vi "Gear Vision Align.vi"(5 "Reinitialize?":bool, 6 "PID gains":T1={"proportional gain (Kc)"=1.0, "integral time (Ti, min)"=0.01, "derivative time (Td, min)"=0.0} {"derivative time (Td, min)" format="%.3f"; "integral time (Ti, min)" format="%.3f"; "proportional gain (Kc)" format="%.3f"}, 7 "Gyro Tolerance":dbl, 8 "X Min":dbl, 9 "X Max":dbl, 10 "Goal Angle Difference":dbl) -> (0 "Finished?":bool, 3 "X Out":dbl)   [LabVIEW 2016]
uses:
  Common Code/PID Gains.ctl
  Robot Global Data.vi
  <vilib>/addons/control/pid/pid.llb/PID (DBL).vi
  <vilib>/addons/control/pid/NI_PID_pid.lvlib
panel:
  out "Heading Target":dbl
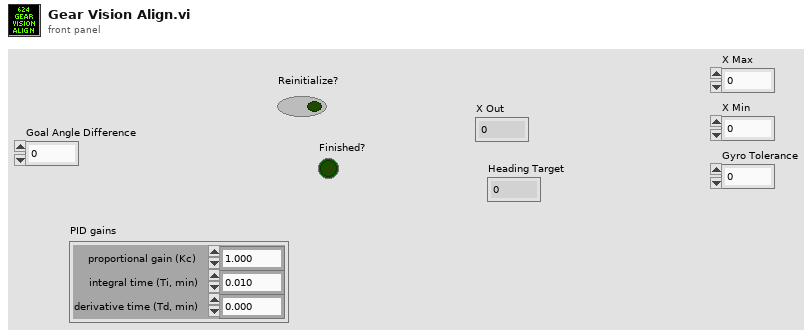
[diagram p1: front panel]
types:
  T1 = typedef "PID Gains.ctl" = cluster{"proportional gain (Kc)":dbl, "integral time (Ti, min)":dbl, "derivative time (Td, min)":dbl}
  T2 = typedef "Drivetrain Status Cluster.ctl" = cluster{"Y (Throttle)":dbl, "X (Steer)":dbl, "Z (Strafe)":dbl, "Heading Target":dbl, "Center Piston Down?":bool, "Traction?":bool, "Gyro Steer Finished?":bool, "Distance Drive Finished?":bool, "Gyro":dbl, "Distance Target":dbl, "Y Max Output":dbl, "Y Min Output":dbl, "X Max Output":dbl, "X Min Output":dbl, "Z Max Output":dbl, "Z Min Output":dbl, "Translation Target":dbl, "Translation Drive Finished?":bool, "PID Auto Drive Finished?":bool, "Brake?":bool, "Vision Aligned?":bool, "Creep Mode Engaged?":bool, "Drivetrain Mode":T3}
  T3 = typedef "Drivetrain Mode.ctl" = enum16{"Gear Vision Align", "Manual", "Gyro Steer", "Distance Drive", "Translate Drive", "Goal Vision Align", "PID Drive"}
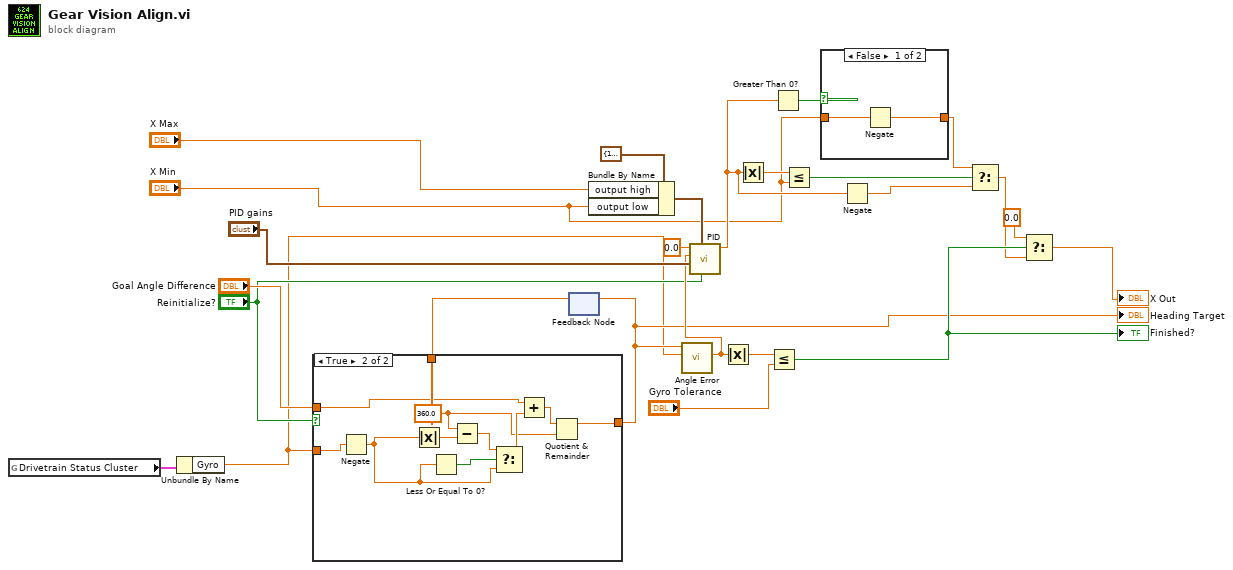
[diagram p0: block diagram]
diagram:
  n1 = global read "Robot Global Data.vi" "Drivetrain Status Cluster"() -> (w11:T2)
  n2 = Unbundle By Name(w11) -> ("Gyro"=w4:dbl)
  n3 = feedback #1() -> (w8:dbl)  [unwired: 1 in]
  n4 = case shown="True" "Reinitialize?" {
    tunnel: [w26 w28] -> w7
    tunnel: "Goal Angle Difference" -> [_ w31]
    tunnel: w8 -> [w26 _]
    tunnel: w4 -> [_ w27]
    frame False {
    }
    frame True {
      w29 = 360.0 ("x")
      n5 = Negate(x=w27) -> (-x=w33:dbl)
      n6 = Absolute Value(x=w33) -> (abs(x)=w35:dbl)
      n7 = Less Or Equal To 0?(x=w33) -> (x <= 0?=w36:bool)
      n8 = Subtract(x=w29, y=w35) -> (x-y=w34:dbl)
      n9 = Select(t=w34, s=w36, f=w33) -> (s? t:f=w32:dbl)
      n10 = Add(x=w31, y=w32) -> (x+y=w30:dbl)
      n11 = Quotient & Remainder(x=w30, y=w29) -> (x-y*floor(x/y)=w28:dbl)  [unwired: 1 out]
    }
  }
  "Heading Target" <- w7
  n12 = feedback-in #1(w7) -> ()
  n13 = Bundle By Name(cluster=cluster{"output high":dbl, "output low":dbl} {"output high"=100.0, "output low"=-100.0} ("output range"), "output high"="X Max", "output low"="X Min") -> (w22:cluster{"output high":dbl, "output low":dbl})
  n14 = call "Angle Error.vi"("Angle"=w4, "Target Angle"=w7) -> ("Error"=w9:dbl)  [unwired: 9 in]
  n15 = call-poly <vilib>:"PID.vi"("reinitialize? (F)"="Reinitialize?", "output range"=w22, "PID gains"="PID gains", "process variable"=w9, "setpoint"=0.0) -> ("output"=w19:dbl)  [unwired: 5 in, 1 out]
  n16 = Absolute Value(x=w9) -> (abs(x)=w18:dbl)
  n17 = Absolute Value(x=w19) -> (abs(x)=w21:dbl)
  n18 = Less Or Equal?(x=w18, y="Gyro Tolerance") -> (x <= y?=w16:bool)
  "Finished?" <- w16
  n19 = Greater Than 0?(x=w19) -> (x > 0?=w3:bool)
  n20 = Less Or Equal?(x=w21, y="X Min") -> (x <= y?=w20:bool)
  n21 = case shown="False" w3 {
    tunnel: "X Min" -> [w38 w39]
    tunnel: [w37 w39] -> w1
    frame False {
      n22 = Negate(x=w38) -> (-x=w37:dbl)
    }
    frame True {
    }
  }
  n23 = Negate(x=w19) -> (-x=w12:dbl)
  n24 = Select(t=w1, s=w20, f=w12) -> (s? t:f=w15:dbl)
  n25 = Select(t=0.0, s=w16, f=w15) -> (s? t:f=→"X Out":dbl)
